vi "TagDefine.vi"(8 "LUT in":string, 11 "Strings In":string[](array[string])) -> (0 "String Out":string, 3 "LUTs out":string[](array[string]))   [LabVIEW 2022 SP3]
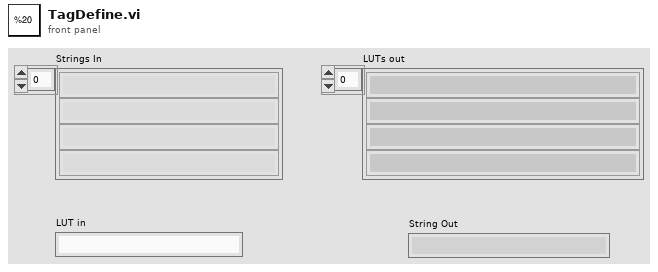
[diagram p1: front panel]
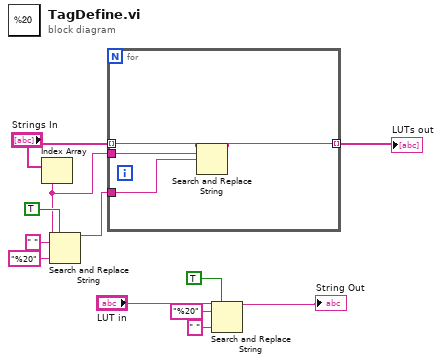
[diagram p0: block diagram]
diagram:
  n1 = Index Array(array="Strings In") -> (element=w2:string)  [unwired: 1 in]
  n2 = Search and Replace String(replace all?=TRUE ("replace all? (F)"), input string=w2, search string=" ", replace string="%20" ("replace string (\"\")")) -> (result string=w1:string)  [unwired: 4 in, 3 out]
  n3 = for {
    tunnel: "Strings In" -> [w16] mode=indexing
    tunnel: [w13] -> w7 mode=indexing
    tunnel: w2 -> [w15]
    tunnel: w1 -> [w14]
    n4 = Search and Replace String(input string=w16, search string=w15, replace string=w14) -> (result string=w13:string)  [unwired: 5 in, 3 out]
  }
  "LUTs out" <- w7
  n5 = Search and Replace String(replace all?=TRUE ("replace all? (F)"), input string="LUT in", search string="%20", replace string=" " ("replace string (\"\")")) -> (result string=→"String Out":string)  [unwired: 4 in, 3 out]
